vi "BTS_PWM Waveform Analysis_GBDC-7.vi"(0 "Analysis Leg":i32, 5 "Active Leg":i32, 7 "Duty Cycle":i32=25, 9 "Waveform":waveform(dbl)[](array[waveform]), 11 "error in (no error)":errorcluster) -> (8 "error out":errorcluster, 10 "Result (Boolean)":bool, 15 "Message":string)   [LabVIEW 2022 SP3]
uses:
  <vilib>/measure/mascope.llb/Pulse Measurements 1 chan.vi
  <vilib>/measure/madcrms.llb/Basic Averaged DC-RMS for 1 Chan.vi
  <vilib>/measure/NI_MAPro.lvlib
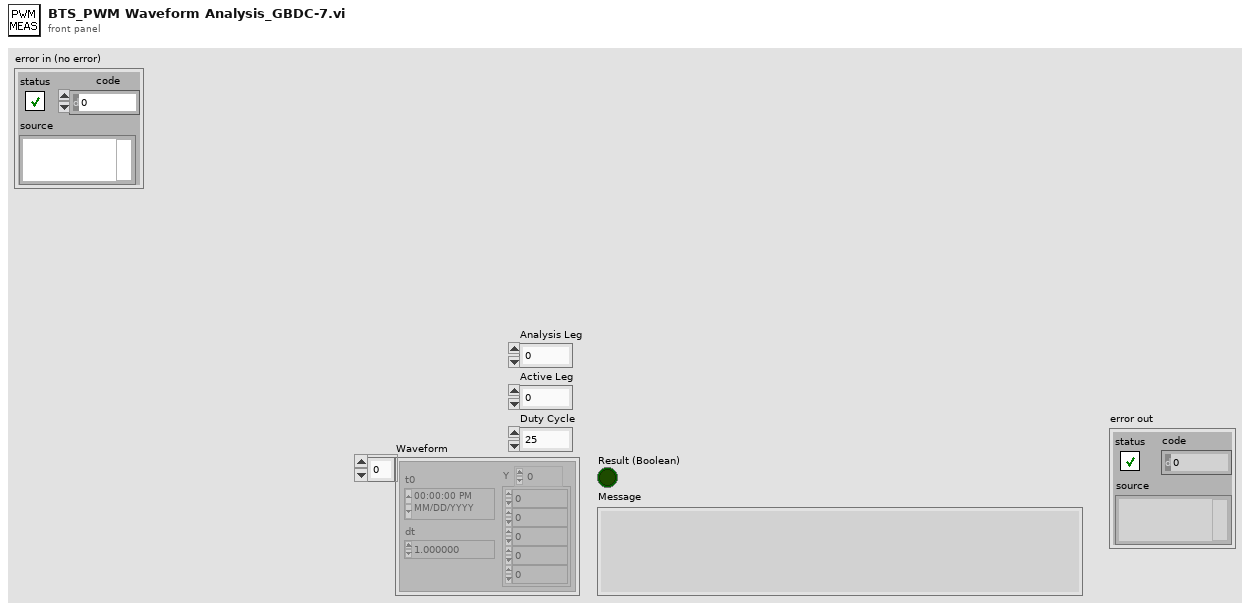
[diagram p1: front panel]
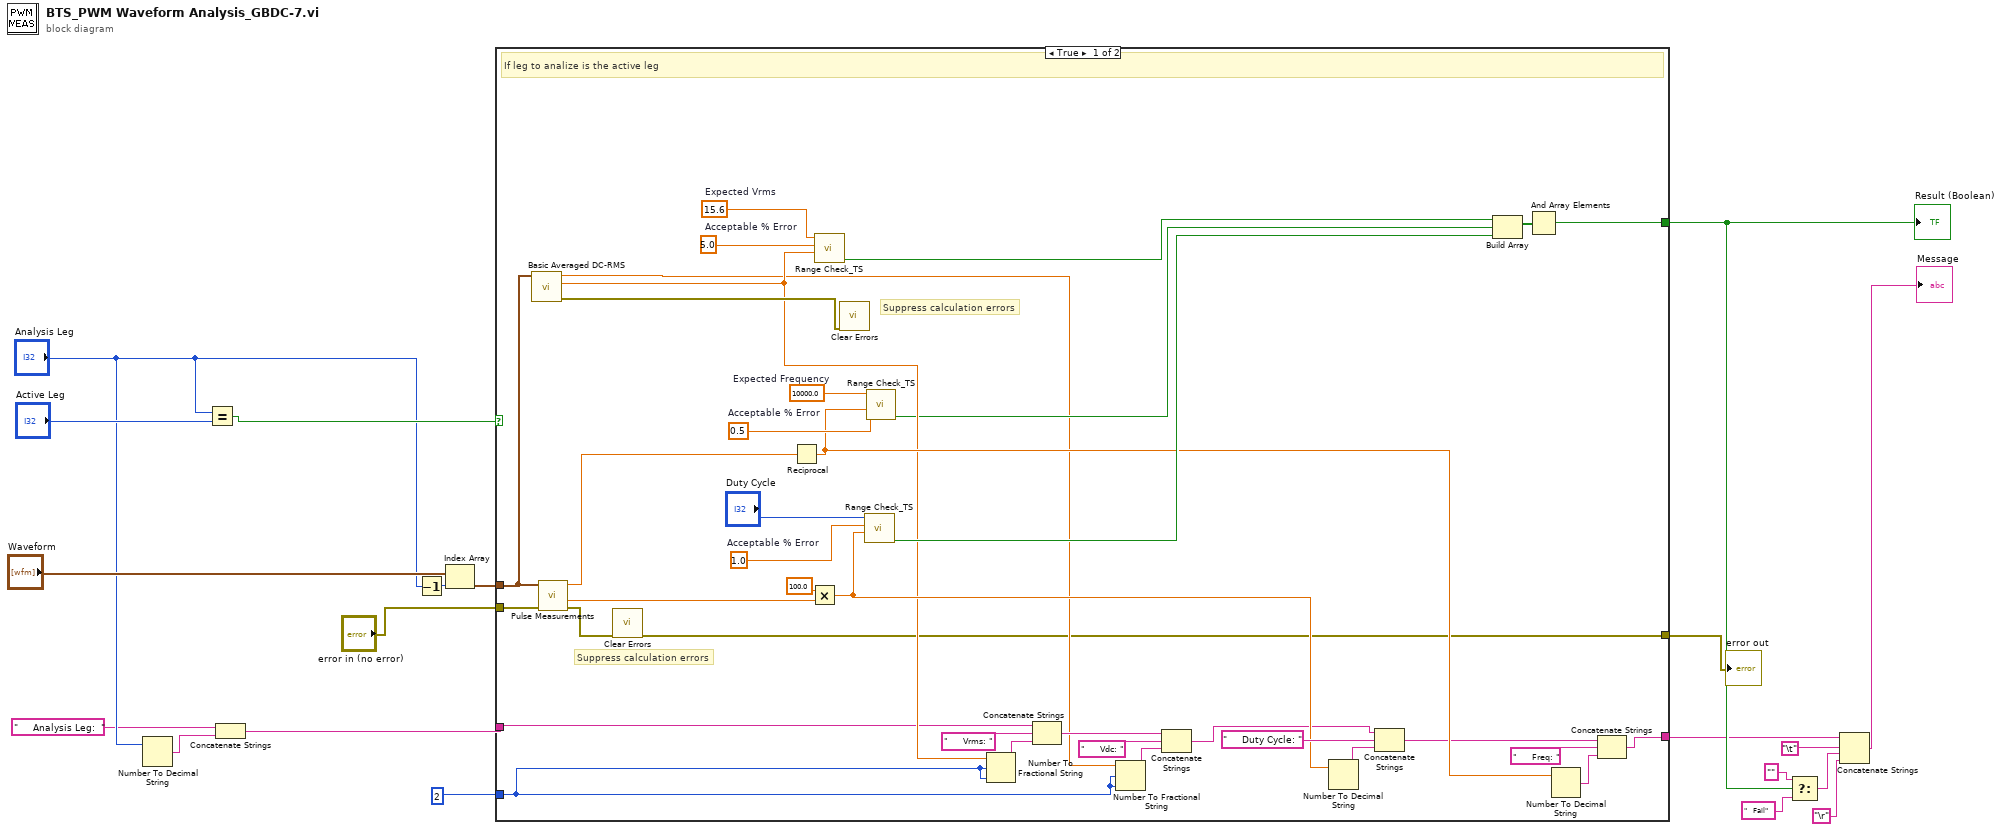
[diagram p0: block diagram]
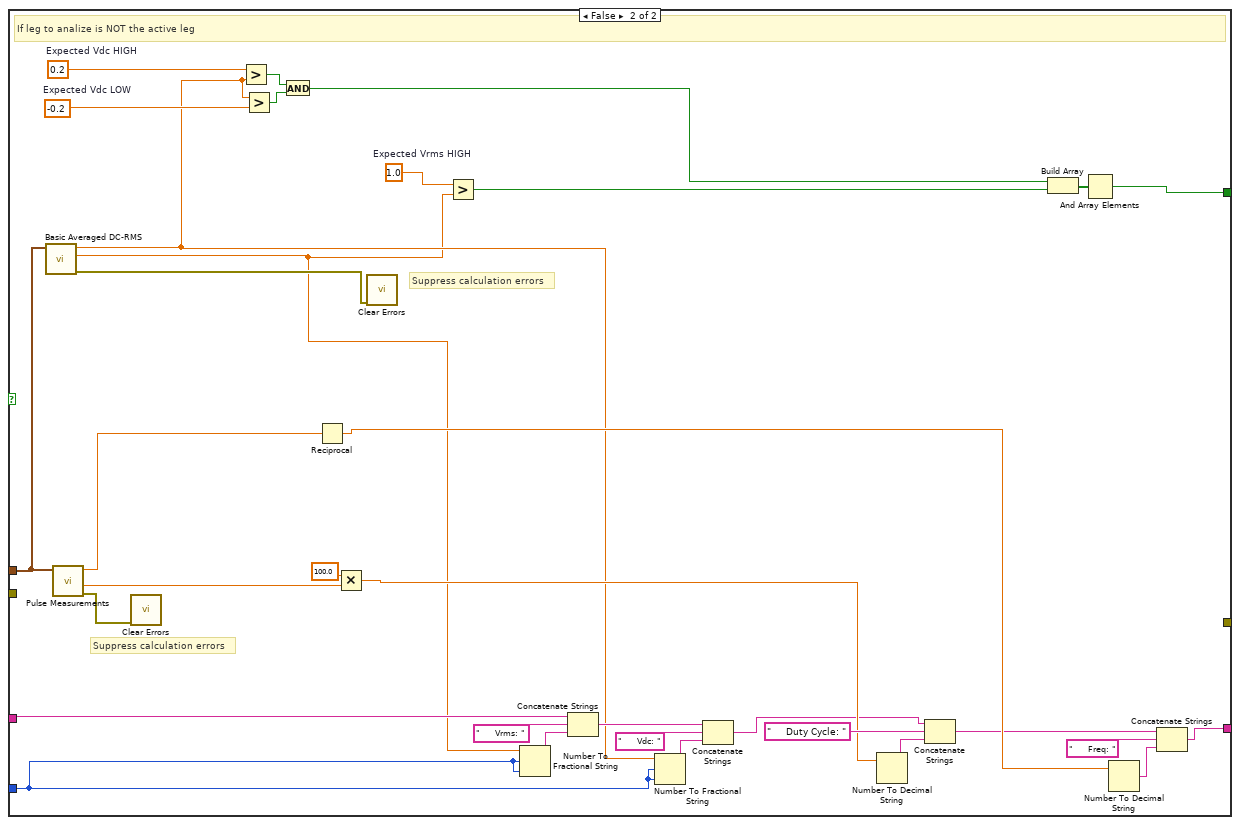
[diagram p2: hidden frame]
diagram:
  n1 = Number To Decimal String(number="Analysis Leg") -> (decimal integer string=w3:string)  [unwired: 1 in]
  n2 = Equal?(x="Analysis Leg", y="Active Leg") -> (x = y?=w7:bool)
  n3 = Concatenate Strings("     Analysis Leg:  ", w3) -> (w4:string)
  n4 = Decrement(x="Analysis Leg") -> (x-1=w20:i32)
  n5 = Index Array(array="Waveform", index=w20) -> (element=w16:waveform(dbl))
  n6 = case shown="True" w7 {
    tunnel: w16 -> [w41 w78]
    tunnel: [w35 w75] -> w12
    tunnel: [w24 w62] -> w11
    tunnel: w4 -> [w26 w64]
    tunnel: 2 -> [w23 w61]
    tunnel: "error in (no error)" -> [w22 _]
    tunnel: [w21 _] -> w1
    frame True {
      w29 = 5.0  # Acceptable % Error
      w28 = 15.6  # Expected Vrms
      w50 = 1.0  # Acceptable % Error
      w51 = 0.5  # Acceptable % Error
      w46 = 10000.0  # Expected Frequency
      # "Suppress calculation errors"
      # "Suppress calculation errors"
      # "If leg to analize is the active leg"
      n7 = call-poly <vilib>:"Basic Averaged DC-RMS.vi"("signal in"=w41) -> ("error out"=w42:errorcluster, "RMS value"=w37:dbl, "DC value"=w27:dbl)  [unwired: 7 in, 1 out]
      n8 = call-poly <vilib>:"Pulse Measurements.vi"("error in (no error)"=w22, "signal in"=w41) -> ("error out"=w52:errorcluster, "duty cycle"=w54:dbl, "period"=w53:dbl)  [unwired: 5 in, 2 out]
      n9 = call <vilib>:"Clear Errors.vi"("error in (no error)"=w52) -> ("error out"=w21:errorcluster)  [unwired: 5 in, 1 out]
      n10 = Reciprocal(x=w53) -> (1/x=w43:dbl)
      n11 = Multiply(x=100.0, y=w54) -> (x*y=w47:dbl)
      n12 = call "Range Check_TS.vi"("Actual Value"=w37, "Acceptable% Error"=w29, "Expected Value"=w28) -> ("Result (Boolean)"=w40:bool)  [unwired: 6 in, 2 out]
      n13 = call <vilib>:"Clear Errors.vi"("error in (no error)"=w42) -> ()  [unwired: 5 in, 2 out]
      n14 = call "Range Check_TS.vi"("Actual Value"=w47, "Acceptable% Error"=w50, "Expected Value"="Duty Cycle") -> ("Result (Boolean)"=w55:bool)  [unwired: 6 in, 2 out]
      n15 = call "Range Check_TS.vi"("Actual Value"=w43, "Acceptable% Error"=w51, "Expected Value"=w46) -> ("Result (Boolean)"=w36:bool)  [unwired: 6 in, 2 out]
      n16 = Number To Fractional String(number=w37, width (-)=w23, precision (6)=w23) -> (F-format string=w39:string)  [unwired: 1 in]
      n17 = Concatenate Strings(w26, "     Vrms: " ("string"), w39) -> (w31:string)
      n18 = Number To Fractional String(number=w27, width (-)=w23, precision (6)=w23) -> (F-format string=w33:string)  [unwired: 1 in]
      n19 = Concatenate Strings(w31, "     Vdc: " ("string"), w33) -> (w25:string)
      n20 = Number To Decimal String(number=w47) -> (decimal integer string=w48:string)  [unwired: 1 in]
      n21 = Concatenate Strings(w25, "     Duty Cycle: " ("string"), w48) -> (w32:string)
      n22 = Build Array(w40, w36, w55) -> (w56:bool[])
      n23 = And Array Elements(Boolean array=w56) -> (logical AND=w35:bool)
      n24 = Number To Decimal String(number=w43) -> (decimal integer string=w44:string)  [unwired: 1 in]
      n25 = Concatenate Strings(w32, "     Freq: " ("string"), w44) -> (w24:string)
    }
    frame False {
      w60 = 1.0  # Expected Vrms HIGH
      w69 = -0.2  # Expected Vdc LOW
      w70 = 0.2  # Expected Vdc HIGH
      # "Suppress calculation errors"
      # "Suppress calculation errors"
      # "If leg to analize is NOT the active leg"
      n26 = call-poly <vilib>:"Basic Averaged DC-RMS.vi"("signal in"=w78) -> ("error out"=w79:errorcluster, "RMS value"=w59:dbl, "DC value"=w65:dbl)  [unwired: 7 in, 1 out]
      n27 = call-poly <vilib>:"Pulse Measurements.vi"("signal in"=w78) -> ("error out"=w86:errorcluster, "duty cycle"=w88:dbl, "period"=w87:dbl)  [unwired: 6 in, 2 out]
      n28 = call <vilib>:"Clear Errors.vi"("error in (no error)"=w86) -> ()  [unwired: 5 in, 2 out]
      n29 = Greater?(x=w70, y=w65) -> (0:w68:bool)
      n30 = Greater?(x=w65, y=w69) -> (0:w67:bool)
      n31 = And(x=w68, y=w67) -> (x .and. y?=w66:bool)
      n32 = Reciprocal(x=w87) -> (1/x=w80:dbl)
      n33 = Multiply(x=100.0, y=w88) -> (x*y=w83:dbl)
      n34 = call <vilib>:"Clear Errors.vi"("error in (no error)"=w79) -> ()  [unwired: 5 in, 2 out]
      n35 = Greater?(x=w60, y=w59) -> (0:w58:bool)
      n36 = Number To Fractional String(number=w59, width (-)=w61, precision (6)=w61) -> (F-format string=w77:string)  [unwired: 1 in]
      n37 = Concatenate Strings(w64, "     Vrms: " ("string"), w77) -> (w71:string)
      n38 = Number To Fractional String(number=w65, width (-)=w61, precision (6)=w61) -> (F-format string=w73:string)  [unwired: 1 in]
      n39 = Concatenate Strings(w71, "     Vdc: " ("string"), w73) -> (w63:string)
      n40 = Number To Decimal String(number=w83) -> (decimal integer string=w84:string)  [unwired: 1 in]
      n41 = Concatenate Strings(w63, "     Duty Cycle: " ("string"), w84) -> (w72:string)
      n42 = Build Array(w66, w58) -> (w89:bool[])
      n43 = And Array Elements(Boolean array=w89) -> (logical AND=w75:bool)
      n44 = Number To Decimal String(number=w80) -> (decimal integer string=w81:string)  [unwired: 1 in]
      n45 = Concatenate Strings(w72, "     Freq: " ("string"), w81) -> (w62:string)
    }
  }
  "Result (Boolean)" <- w12
  "error out" <- w1
  n46 = Select(t="" ("string"), s=w12, f="   Fail" ("string")) -> (s? t:f=w13:string)
  n47 = Concatenate Strings(w11, "\t", w13, "\r") -> (→"Message":string)
